vi "Offset Widget Transaction Lists.vi"(7 "Offset Type":T5, 8 "error in (no error)":errorcluster, 9 "Coordinate Space":bool caption="Coord", 10 "Rigid Connection":bool, 11 "Number of\nLBCBs":T6) -> (0 "error out":errorcluster, 2 "Transactions":T2[](array[typedef]))   [LabVIEW 2013]
uses:
  Global Data/Transactions/Dataset Source.ctl
  Global Data/Transactions/Dataset Type.ctl
  Apps/Yes No Button.ctl
  Global Data/Transactions/Dataset Transaction Id.ctl
  Data Access Objects/Application/Number Of LBCBs.ctl
  Offsets/Offset Types.ctl
panel:
  in  "Cartesian Types":T1[](array[typedef])=[enum."Displacement Command", enum."Displacement", enum."Force"]
  in  "Actuator Types":T1[](array[typedef])=[enum."Actuator Command", enum."LVDT", enum."Load Cell"]
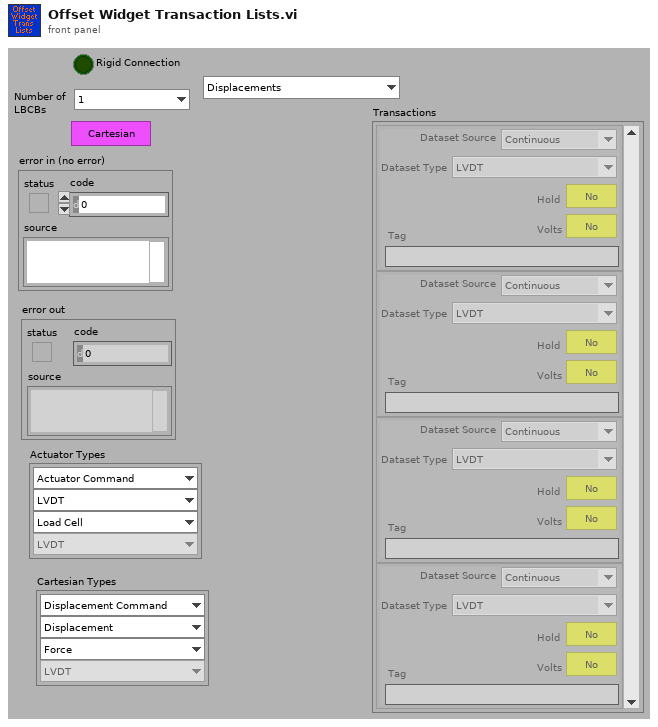
[diagram p1: front panel]
types:
  T1 = typedef "Dataset Type.ctl" = enum16{"LVDT", "Load Cell", "Actuator Command", "Servo Error", "Displacement Command", "Displacement", "Force"}
  T2 = typedef "Dataset Transaction Id.ctl" = cluster{"Dataset Source":T3, "Dataset Type":T1, "Hold":T4, "Volts":T4, "Tag":string}
  T3 = typedef "Dataset Source.ctl" = enum16{"Continuous", "Hold", "ED", "Volts", "Offsets"}
  T4 = typedef "Yes No Button.ctl" = bool
  T5 = typedef "Offset Types.ctl" = enum16{"Displacements", "Forces", "External Sensors"}
  T6 = typedef "Number Of LBCBs.ctl" = enum16{"1", "2"}
  T7 = typedef "Dataset Source.ctl" = enum16{"LBCB 1", "LBCB 2", "Combined", "External Sensors"}
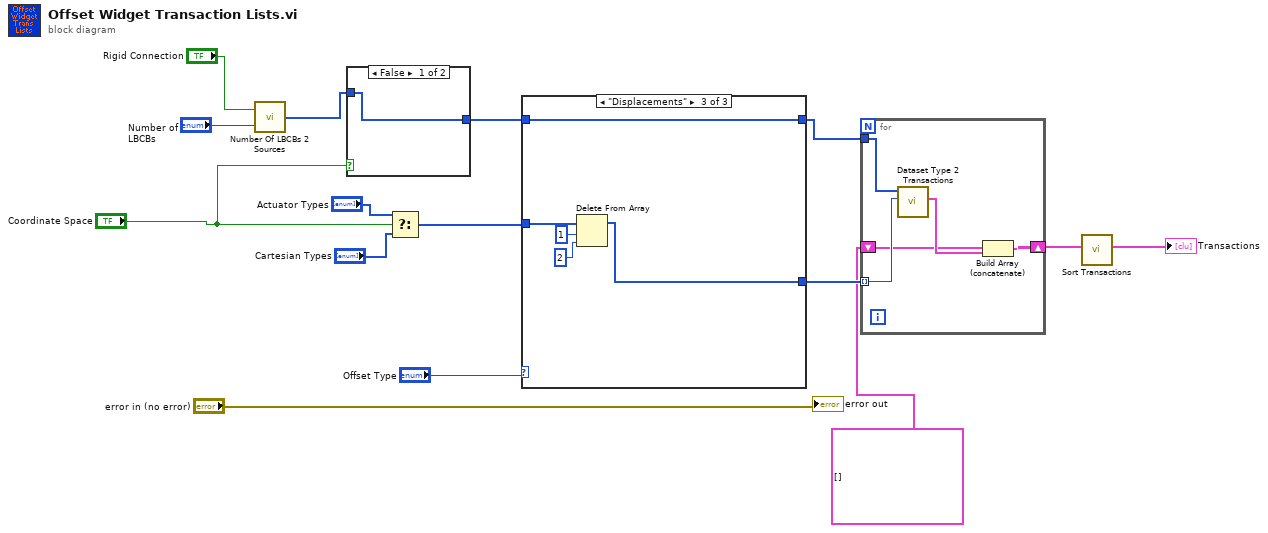
[diagram p0: block diagram]
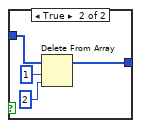
[diagram p2: hidden frame]
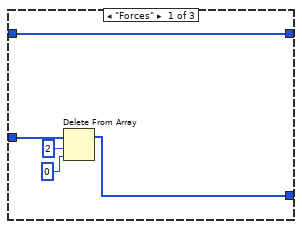
[diagram p3: hidden frame]
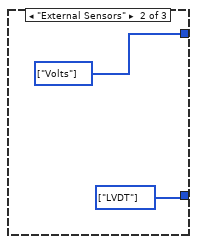
[diagram p4: hidden frame]
diagram:
  n1 = call "Number Of LBCBs 2 Sources.vi"("Number of LBCBs"="Number of\nLBCBs", "Combined LBCBs"="Rigid Connection") -> ("Sources"=w3:T7[])
  n2 = case shown="False" "Coordinate Space" {
    tunnel: w3 -> [w16 w20]
    tunnel: [w16 w19] -> w2
    frame False {
    }
    frame True {
      n3 = Delete From Array(array=w20, length=1, index=2) -> (array with subset deleted=w19:T7[])  [unwired: 1 out]
    }
  }
  n4 = Select(t="Actuator Types", s="Coordinate Space", f="Cartesian Types") -> (s? t:f=w9:T1[])
  n5 = case shown="\"Displacements\"" "Offset Type" {
    tunnel: w9 -> [w25 _ w32]
    tunnel: w2 -> [w21 _ w28]
    tunnel: [w22 w27 w29] -> w8
    tunnel: [w21 w26 w28] -> w7
    frame "Forces" {
      n6 = Delete From Array(array=w25, length=2, index=0) -> (array with subset deleted=w22:T1[])  [unwired: 1 out]
    }
    frame "External Sensors" {
      w26 = T3[] [enum."Volts"] items=["Continuous", "Hold", "ED", "Volts", "Offsets"] ("Sources")
      w27 = T1[] [enum."LVDT"] items=["LVDT", "Load Cell", "Actuator Command", "Servo Error", "Displacement Command", "Displacement", "Force"] ("Types")
    }
    frame "Displacements" {
      n7 = Delete From Array(array=w32, length=1, index=2) -> (array with subset deleted=w29:T1[])  [unwired: 1 out]
    }
  }
  n8 = for {
    tunnel: w8 -> [w36] mode=indexing
    tunnel: w7 -> [w37]
    shift-right: [w34] -> w6
    shift-left: T2[] [] -> [w33]
    n9 = call "Dataset Type 2 Transactions.vi"("Dataset Type"=w36, "Sources"=w37) -> ("Transactions"=w35:T2[])  [unwired: 9 in]
    n10 = Build Array (concatenate)(w33, w35) -> (w34:T2[])
  }
  n11 = call "Sort Transactions.vi"("Transactions In"=w6) -> ("Transactions Out"=→"Transactions":T2[])  [unwired: 10 in]
  "error out" <- "error in (no error)"
